vi "Verify with 3 Scrubbers.vi"(8 "error in":errorcluster) -> (0 "error out":errorcluster)   [LabVIEW 2020, in "Scrubber Testing.lvclass"]
uses:
  Scrubber Testing.lvclass
  Scrubber Testing.lvclass/Scrubber Testing.ctl
  <vilib>/addons/_JKI Toolkits/Caraya/classes/Test/Test.lvclass
  4b862e9e-fcb2-487f-ab73-d9f83fbf4d2c.vi
  Source/Approval Tests/Regex Scrubber/Regex Scrubber.lvclass
  Source/Approval Tests/Options/Options.lvclass
  C:/Users/SAS/Desktop/ApprovalTests.LabVIEW/Source/Approval Tests/Regex Scrubber/Regex Scrubber.lvclass
  C:/Users/SAS/Desktop/ApprovalTests.LabVIEW/Source/Approval Tests/Scrubber/Scrubber.lvclass
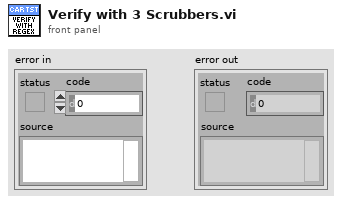
[diagram p1: front panel]
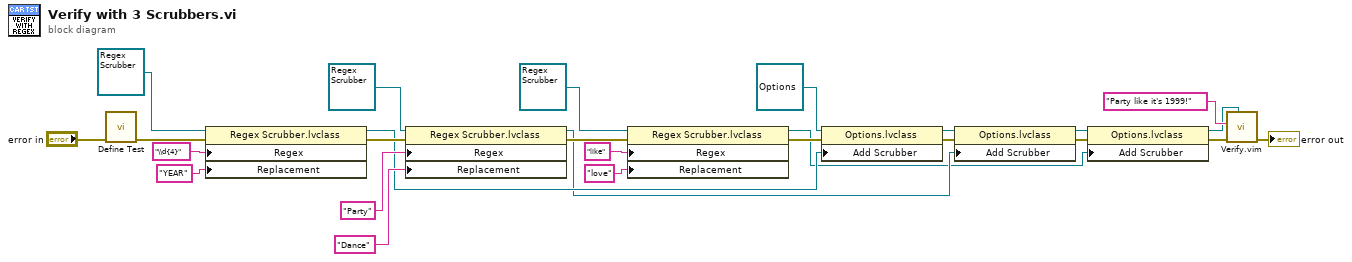
[diagram p0: block diagram]
diagram:
  n1 = call <vilib>:"Define Test.vi"("error in (no error)"="error in") -> ("error out"=w26:errorcluster)  [unwired: 9 in, 1 out]
  n2 = property class="Regex Scrubber.lvclass"(reference=refnum<class "Regex Scrubber.lvclass"> refnum ("Approval Tests.lvlib:Regex Scrubber.lvclass"), error in=w26, "Regex"="\\d{4}", "Replacement"="YEAR") -> (reference out=w9:refnum<class "Regex Scrubber.lvclass">, error out=w23:errorcluster)
  n3 = property class="Regex Scrubber.lvclass"(reference=refnum<class "Regex Scrubber.lvclass"> refnum ("Approval Tests.lvlib:Regex Scrubber.lvclass"), error in=w23, "Regex"="Party", "Replacement"="Dance") -> (reference out=w7:refnum<class "Regex Scrubber.lvclass">, error out=w22:errorcluster)
  n4 = property class="Regex Scrubber.lvclass"(reference=refnum<class "Regex Scrubber.lvclass"> refnum ("Approval Tests.lvlib:Regex Scrubber.lvclass"), error in=w22, "Regex"="like", "Replacement"="love") -> (reference out=w1:refnum<class "Regex Scrubber.lvclass">, error out=w18:errorcluster)
  n5 = property class="Options.lvclass"(reference=refnum<class "Options.lvclass"> refnum ("Approval Tests.lvlib:Options.lvclass"), error in=w18, "Add Scrubber"=w9) -> (reference out=w8:refnum<class "Options.lvclass">, error out=w21:errorcluster)
  n6 = property class="Options.lvclass"(reference=w8, error in=w21, "Add Scrubber"=w7) -> (reference out=w6:refnum<class "Options.lvclass">, error out=w20:errorcluster)
  n7 = property class="Options.lvclass"(reference=w6, error in=w20, "Add Scrubber"=w1) -> (reference out=w5:refnum<class "Options.lvclass">, error out=w19:errorcluster)
  n8 = call "Verify.vim"("Options"=w5, "error in"=w19, "Test Data"="Party like it's 1999!") -> ("error out"=→"error out":errorcluster)  [unwired: 8 in]
